vi "WPI_CameraSet Numeric Appearance Property.vi"(8 "error in (no error)":errorcluster, 9 "Value":i32, 10 "Property Name":string, 11 "CameraDevRef":T1) -> (0 "error out":errorcluster, 3 "CameraDevRef out":T1)   [LabVIEW 2017]
doc: "This software is licensed. Open the labview\\readme\\WPI Robotics Library Open Source License.txt file for more information."
uses:
  <vilib>/Rock Robotics/WPI/Camera/WPI_CameraDevRef.ctl
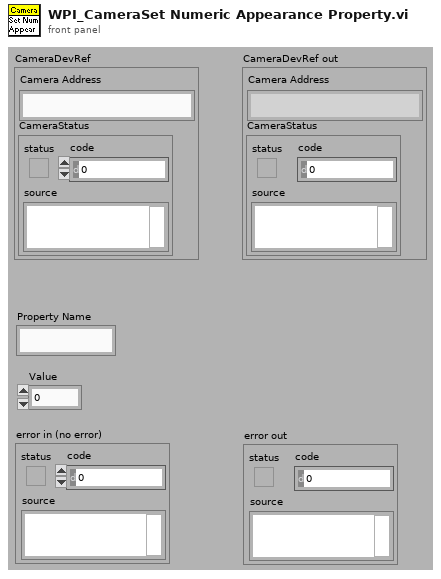
[diagram p1: front panel]
types:
  T1 = typedef "WPI_CameraDevRef.ctl" = cluster{"Camera Address":string, "CameraStatus":errorcluster}
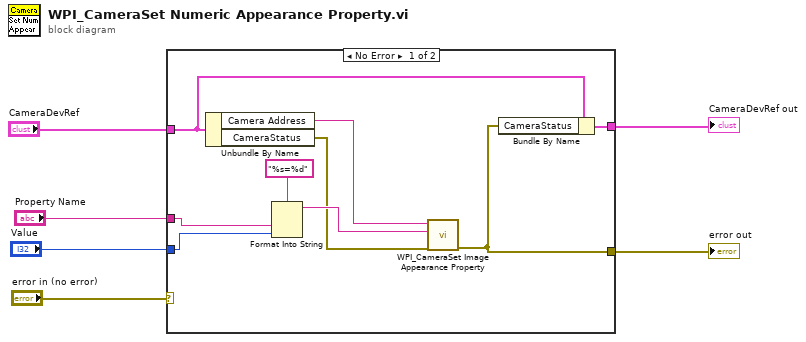
[diagram p0: block diagram]
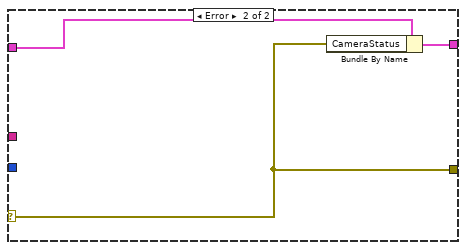
[diagram p2: hidden frame]
diagram:
  n1 = case shown="No Error" "error in (no error)" {
    selector: "error in (no error)" -> [_ w16]
    tunnel: [w15 w16] -> w6
    tunnel: "CameraDevRef" -> [w14 w17]
    tunnel: [w13 w18] -> w4
    tunnel: "Property Name" -> [w12 _]
    tunnel: "Value" -> [w11 _]
    frame No Error {
      n2 = Unbundle By Name(w14) -> ("Camera Address"=w7:string, "CameraStatus"=w8:errorcluster)
      n3 = Format Into String(format string="%s=%d", w12, w11) -> (resulting string=w9:string)  [unwired: 2 in, 1 out]
      n4 = call <vilib>:"WPI_CameraSet Image Appearance Property.vi"("error in"=w8, "Prop String"=w9, "address"=w7) -> ("error out"=w15:errorcluster)  [unwired: 1 in, 7 out]
      n5 = Bundle By Name(cluster=w14, "CameraStatus"=w15) -> (w13:T1)
    }
    frame Error {
      n6 = Bundle By Name(cluster=w17, "CameraStatus"=w16) -> (w18:T1)
    }
  }
  "error out" <- w6
  "CameraDevRef out" <- w4
